vi "niScope Multi Fetch Measurement.vi"(0 "instrument handle":refnum<k15>, 1 "timeout":dbl=5.0 format="%.2f", 5 "channels":string="0", 7 "scalar measurement":T1=4000 items=["None"=4000, "Frequency"=2, "Average Frequency"=1016, "FFT Frequency"=1008, "Period"=3, "Average Period"=1015, "Rise Time"=0, "Fall Time"=1, "Rising Slew Rate"=1010, "Falling Slew Rate"=1011, "Overshoot"=18, "Preshoot"=19, "Voltage RMS"=4, "Voltage Cycle RMS"=16, "AC Estimate"=1012, "FFT Amplitude"=1009, "Voltage Average"=10, "Voltage Cycle Average"=17, "DC Estimate"=1013, "Voltage Max"=6, "Voltage Min"=7, "Voltage Peak-to-Peak"=5, "Voltage High"=8, "Voltage Low"=9, "Voltage Amplitude"=15, "Voltage Top"=1007, "Voltage Base"=1006, "Voltage Base-to-Top"=1017, "Negative Width"=11, "Positive Width"=12, "Negative Duty Cycle"=13, "Positive Duty Cycle"=14, "Integral"=1005, "Area"=1003, "Cycle Area"=1004, "Time Delay"=1014, "Phase Delay"=1018, "Low Ref Volts"=1000, "Mid Ref Volts"=1001, "High Ref Volts"=1002, "Volt. Hist. Mean"=2000, "Volt. Hist. Stdev"=2001, "Volt. Hist. Median"=2003, "Volt. Hist. Mode"=2010, "Volt. Hist. Max"=2005, "Volt. Hist. Min"=2006, "Volt. Hist. Peak-to-Peak"=2002, "Volt. Hist. Mean + Stdev"=2007, "Volt. Hist. Mean + 2 Stdev"=2008, "Volt. Hist. Mean + 3 Stdev"=2009, "Volt. Hist. Hits"=2004, "Volt. Hist. New Hits"=2011, "Time Hist. Mean"=3000, "Time Hist. Stdev"=3001, "Time Hist. Median"=3003, "Time Hist. Mode"=3010, "Time Hist. Max"=3005, "Time Hist. Min"=3006, "Time Hist. Peak-to-Peak"=3002, "Time Hist. Mean + Stdev"=3007, "Time Hist. Mean + 2 Stdev"=3008, "Time Hist. Mean + 3 Stdev"=3009, "Time Hist. Hits"=3004, "Time Hist. New Hits"=3011], 11 "error in":errorcluster) -> (4 "instrument handle out":refnum<k15>, 6 "results":dbl[](array[numeric]) format="%.2f", 15 "error out":errorcluster)   [LabVIEW 2013]
doc: "Fetches a waveform from the digitizer and performs the specified waveform measurement. Use this function for multiple channel and multiple record acquisitions."
uses:
  <instrlib>/niScope/Controls/niScope scalar measurement.ctl
  niScope_32.dll
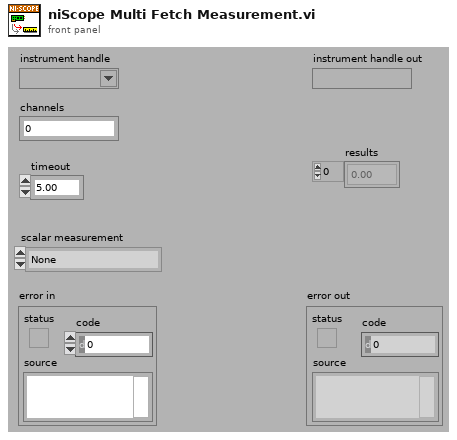
[diagram p1: front panel]
types:
  T1 = typedef "niScope scalar measurement.ctl" = i32
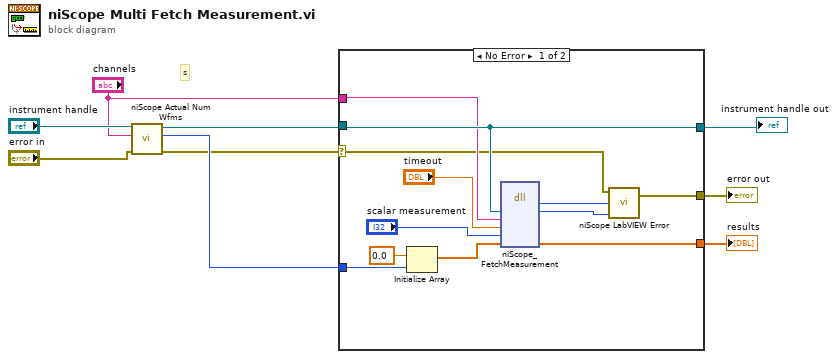
[diagram p0: block diagram]
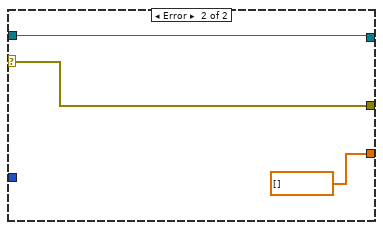
[diagram p2: hidden frame]
diagram:
  # "s"
  n1 = call <instrlib>:"niScope Actual Num Wfms.vi"("error in"="error in", "channels"="channels", "instrument handle"="instrument handle") -> ("error out"=w1:errorcluster, "actual num wfms"=w3:i32, "instrument handle out"=w5:refnum<k15>)  [unwired: 6 in]
  n2 = case shown="No Error" w1 {
    selector: w1 -> [w10 w22]
    tunnel: [w21 w22] -> w9
    tunnel: [w13 dbl[] [] ("measurements")] -> w7
    tunnel: w5 -> [w17 w23]
    tunnel: [w17 w23] -> w8
    tunnel: w3 -> [w16 _]
    tunnel: "channels" -> [w15 _]
    frame No Error {
      n3 = Initialize Array(0.0 ("Element Data"), w16) -> (w14:dbl[])
      n4 = dll-call lib="niScope_*.*" fn="niScope_FetchMeasurement"("instrument handle"=w17, "channelList"=w15, "timeout"="timeout", "scalarMeasFunction"="scalar measurement", "results"=w14) -> ("status"=w20:i32, "instrument handle"=w19:u32, "results"=w13:dbl[])  [unwired: 6 in, 2 out]
      n5 = call <instrlib>:"niScope LabVIEW Error.vi"("instrument handle"=w19, "niScope error code (0)"=w20, "error in (no error)"=w10) -> ("error out"=w21:errorcluster)  [unwired: 2 in]
    }
    frame Error {
    }
  }
  "instrument handle out" <- w8
  "error out" <- w9
  "results" <- w7
